vi "data_load_display_trend_fft_mea_coll_v3.vi"() -> ()   [LabVIEW 2020]
uses:
  <vilib>/Analysis/2dsp.llb/Real FFT.vi
  <vilib>/Utility/file.llb/Read Delimited Spreadsheet (DBL).vi
  <vilib>/Utility/file.llb/Read Delimited Spreadsheet (string).vi
  <vilib>/ptbypt/NI_PtbyPt.lvlib
  <vilib>/Analysis/NI_AALPro.lvlib
  <vilib>/rvi/Analysis/host/Public/NI_FpgaMspHost.lvlib
panel:
  out "Waveform Graph":dbl[][](graph)
  out "XY Graph":cluster{dbl[], dbl[]}(graph)
  out "restored signal":dbl[](array[numeric])
  out "plot restored signal":dbl[](graph)
  out "ploted signal from each selected frequency":dbl[][](graph)
  out "signal from each selected frequency":dbl[][](array[numeric])
  out "phase":dbl[](array[numeric])
  out "magnitude":dbl[](array[numeric])
  out "phase":dbl format="%0.2f"
  out "magnitude":dbl format="%0.2f"
  out "magnitude plot":dbl[](graph)
  out "phase plot":dbl[](graph)
  out "magnitudes":dbl[](array[numeric])
  out "phasees":dbl[](array[numeric])
  out "df (Hz)":dbl
  out "size(s)":i32
  out "xf (frequency)":dbl[](array[numeric])
  in  "decimating factor":i32=3
  out "xf (sample Vs frequency )":dbl[][](array[numeric]) format="%#20_5g"
  out "Imaginary values":dbl[](array[numeric])
  out "real  values":dbl[](array[numeric])
  out "real plot":dbl[](graph)
  out "imaginary plot":dbl[](graph)
  out "Time Domain sequence":cluster{i32, dbl, dbl[]}(graph)
  out "Frequency Interval: delta(f)":dbl
  out "Spectrum plot":cluster{i32, dbl, "spectrum out":dbl[]}(graph)
  out "Remove trend":cluster{"all rows":dbl[], dbl[]}(graph)
  out "Time vs Acceleration  find trend graph":T1(graph)
  out "array w/ subset deleted":dbl[][](array[numeric])
  out "first row":string[][](array[string])
  out "time":dbl[](array[numeric])
  out "Acceleration":dbl[](array[numeric])
  out "Time vs Acceleration graph":cluster{"all rows":dbl[], "all rows":dbl[]}(graph)
  out "stripped path":path
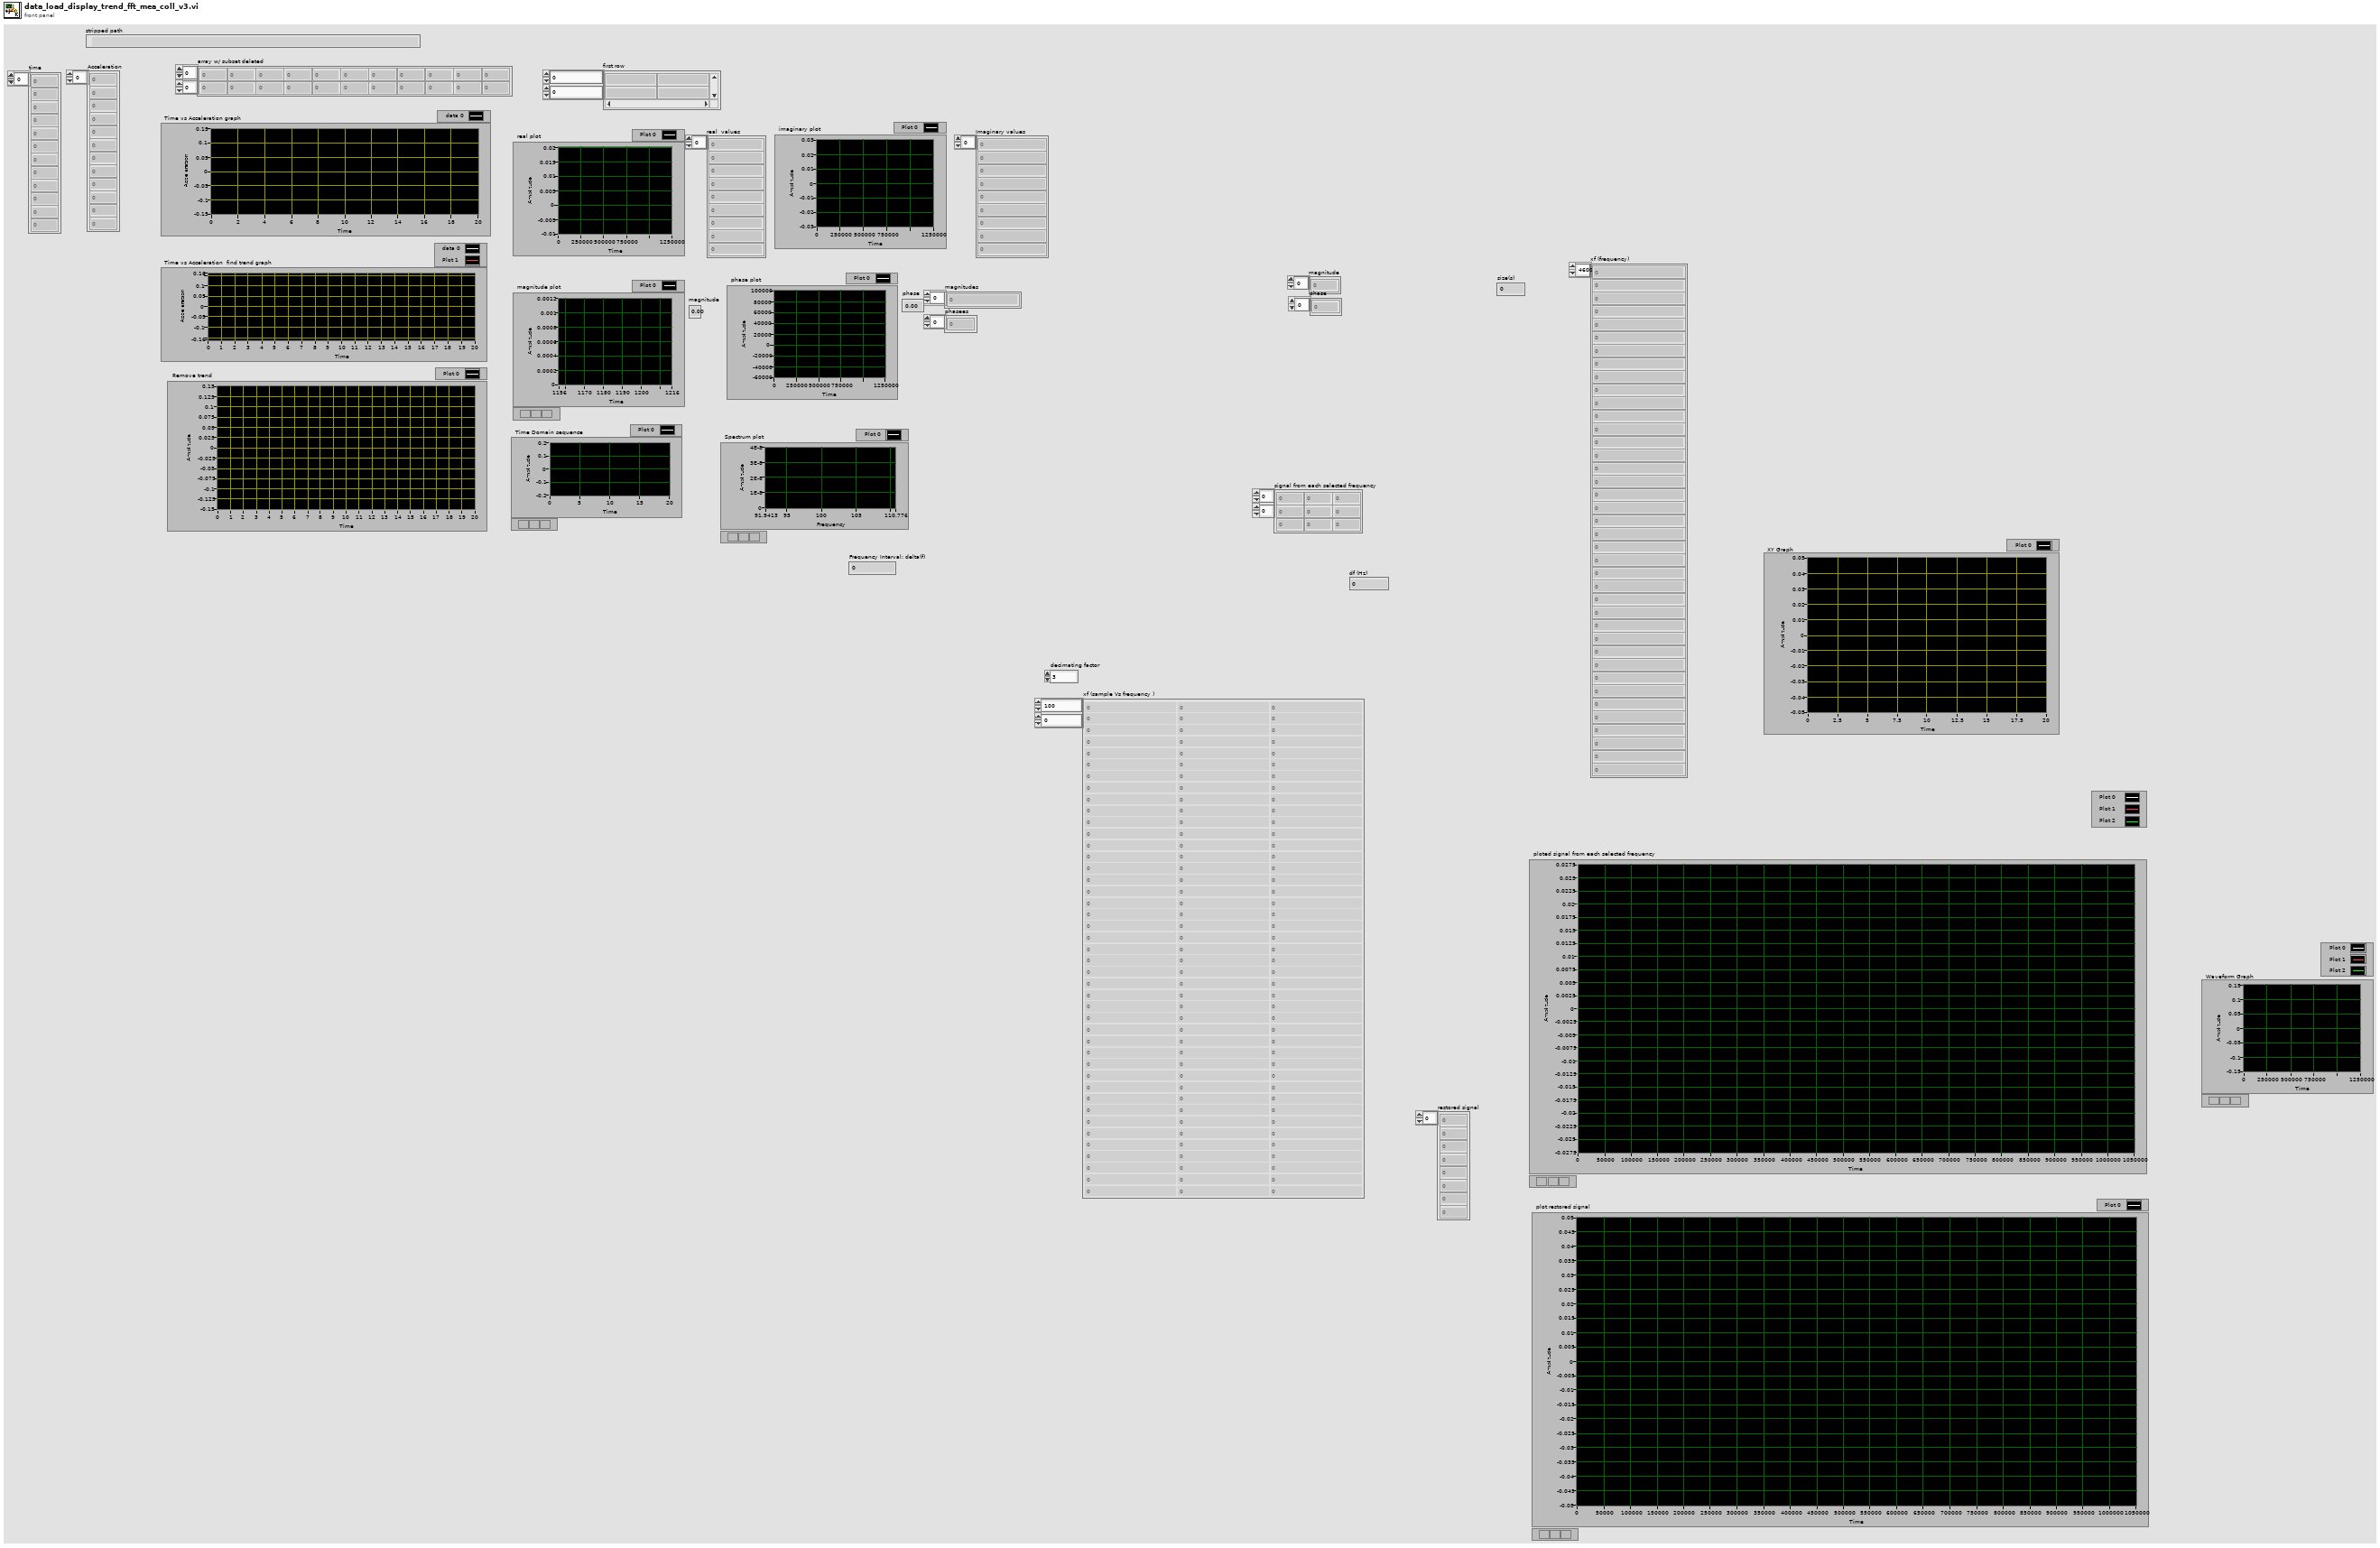
[diagram p1: front panel]
types:
  T1 = cluster{"all rows":dbl[], "Best Linear Fit":dbl[]}
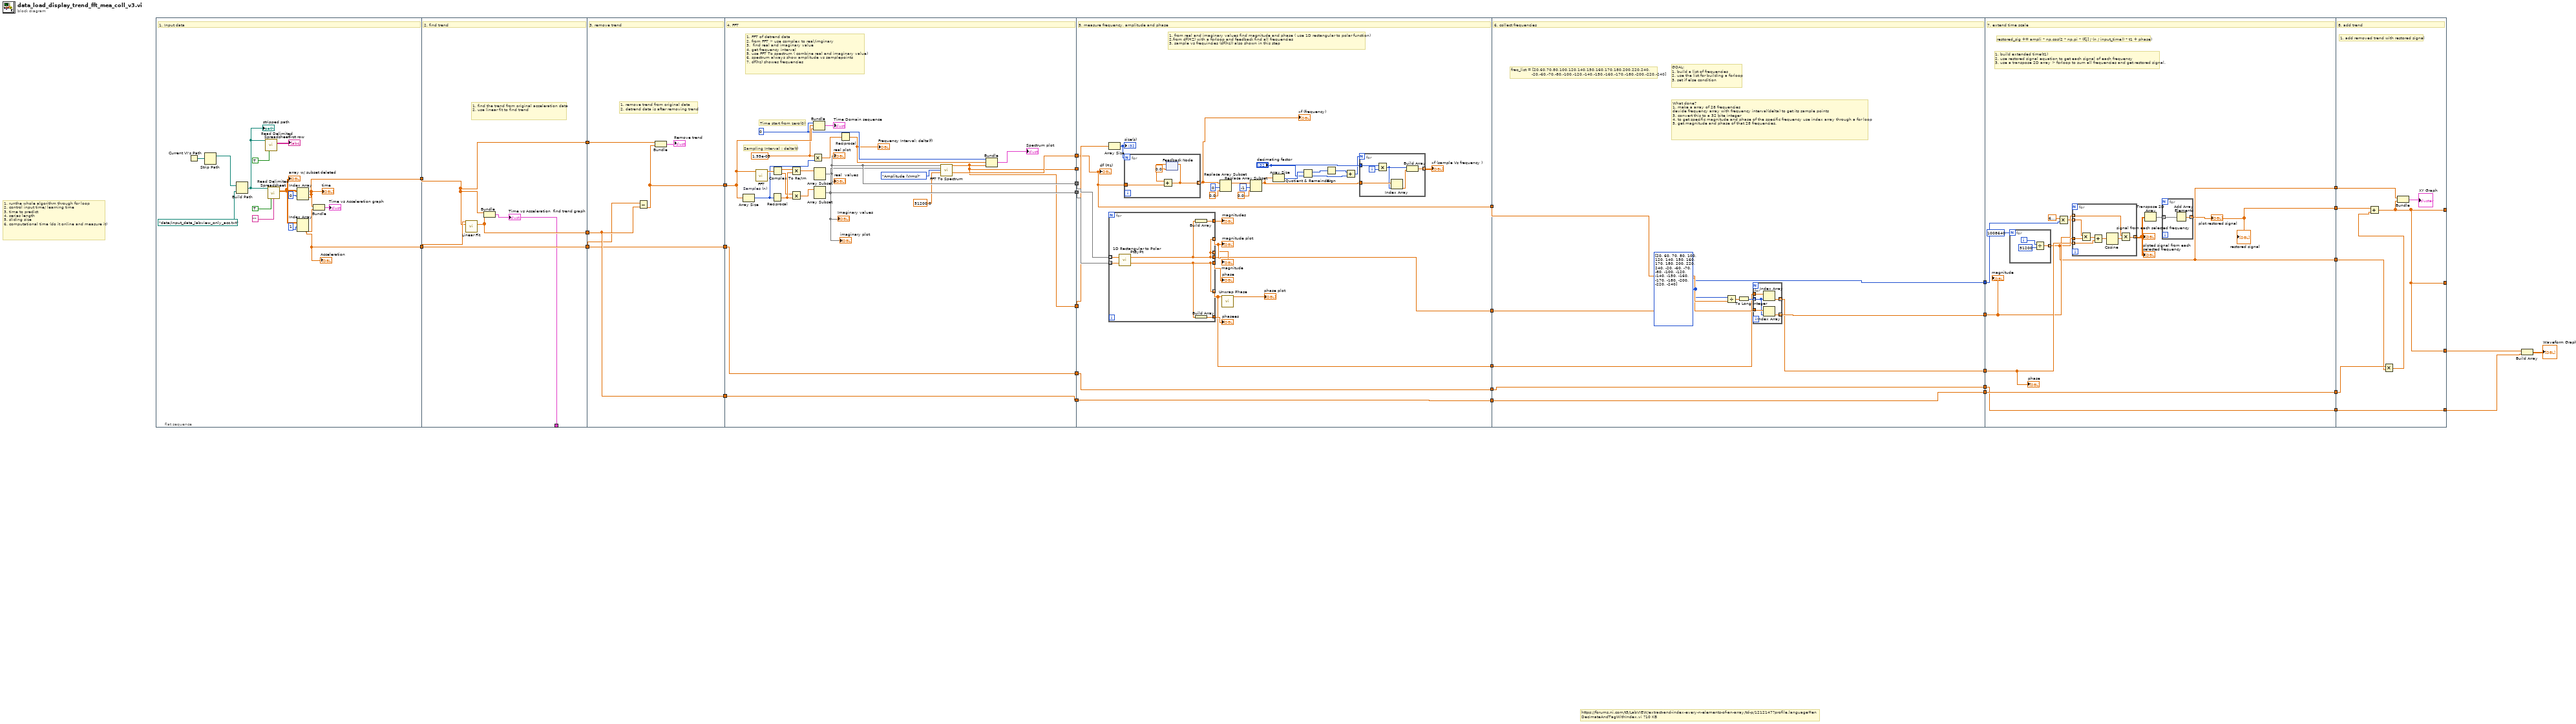
[diagram p0: block diagram]
diagram:
  # "1. runthe whole algorithm through for loop \n2. control input time/ learning time\n3. time to predict\n4. series length\n5. sliding size\n6. computational time (do it online and measure it)"
  # "https://forums.ni.com/t5/LabVIEW/extract-and-index-every-n-elements-of-an-array/td-p/1212147?profile.language=en\nDecimateAndTagWithIndex.vi ?10 KB"
  n1 = flat-sequence {
    tunnel: [w35] -> w33
    tunnel: [w34] -> w32
    tunnel: w33 -> [w50]
    tunnel: [w51] -> w31
    tunnel: [w50] -> w30
    tunnel: [w49] -> w29
    tunnel: w32 -> [w49]
    tunnel: [w48] -> _
    tunnel: w31 -> [w53]
    tunnel: w30 -> [w52]
    tunnel: w29 -> [w56]
    tunnel: [w55] -> w28
    tunnel: [w53] -> w27
    tunnel: [w52] -> w8
    tunnel: w28 -> [w72]
    tunnel: [w69] -> w26
    tunnel: [w68] -> w25
    tunnel: [w60] -> w24
    tunnel: [w61] -> w23
    tunnel: [w60] -> w22
    tunnel: [w58] -> w21
    tunnel: w27 -> [w58]
    tunnel: w8 -> [w57]
    tunnel: [w57] -> w7
    tunnel: w26 -> [w106]
    tunnel: w25 -> [w105]
    tunnel: w24 -> [_]
    tunnel: w23 -> [w84]
    tunnel: w22 -> [w99]
    tunnel: [w84] -> w20
    tunnel: [w83] -> w19
    tunnel: [w81] -> w18
    tunnel: [w80] -> w17
    tunnel: w21 -> [w80]
    tunnel: w7 -> [w79]
    tunnel: [w79] -> w6
    tunnel: w20 -> [w132]
    tunnel: [w129] -> w16
    tunnel: w19 -> [w128]
    tunnel: w18 -> [w127]
    tunnel: [w126] -> w15
    tunnel: [w125] -> w14
    tunnel: [w124] -> w13
    tunnel: w17 -> [w124]
    tunnel: w6 -> [w123]
    tunnel: [w123] -> w5
    tunnel: w16 -> [w147]
    tunnel: w15 -> [w148]
    tunnel: w14 -> [w143]
    tunnel: [w141] -> w12
    tunnel: [w140] -> w11
    tunnel: w13 -> [w140]
    tunnel: [w139] -> w10
    tunnel: [w139] -> w9
    tunnel: w5 -> [w138]
    tunnel: [w138] -> w4
    tunnel: w12 -> [w170]
    tunnel: w11 -> [w168]
    tunnel: w10 -> [w169]
    tunnel: w9 -> [w167]
    tunnel: [w164] -> _
    tunnel: [w165] -> w2
    tunnel: w4 -> [w165]
    tunnel: [w164] -> _
    tunnel: [w164] -> w3
    frame #0 {
      # "1. Input data"
      n2 = Current VI's Path() -> (path=w39:path)
      n3 = Strip Path(path=w39) -> (stripped path=w38:path)  [unwired: 1 out]
      n4 = Build Path(base path=w38, name or relative path=path "data/input_data_labview_only_acc.txt") -> (appended path=w36:path)
      "stripped path" <- w36
      n5 = call-poly <vilib>:"Read Delimited Spreadsheet.vi"("file path (dialog if empty)"=w36, "transpose? (F)"=TRUE) -> ("all rows"=→"first row":string[][])  [unwired: 8 in, 5 out]
      n6 = call-poly <vilib>:"Read Delimited Spreadsheet.vi"("file path (dialog if empty)"=w36, "transpose? (F)"=TRUE, "delimiter (\\t)"="" ("delimiter (\\t)")) -> ("all rows"=w41:dbl[][])  [unwired: 7 in, 5 out]
      "array w/ subset deleted" <- w41
      n7 = Index Array(array=w41, index (row)=0) -> (element=w34:dbl[])  [unwired: 1 in]
      "time" <- w34
      n8 = Index Array(array=w41, index (row)=1) -> (element=w35:dbl[])  [unwired: 1 in]
      "Acceleration" <- w35
      n9 = Bundle("all rows"=w34, "all rows"=w35) -> (→"Time vs Acceleration graph":cluster{"all rows":dbl[], "all rows":dbl[]})  [unwired: 1 in]
    }
    frame #1 {
      # "1. find the trend from original acceleration data\n2. use linear fit to find trend"
      # "2. find trend"
      n10 = call <vilib>:"Linear Fit.vi"("Y"=w50, "X"=w49) -> ("Best Linear Fit"=w51:dbl[])  [unwired: 9 in, 4 out]
      n11 = Bundle("all rows"=w49, "Best Linear Fit"=w51) -> (w48:T1)  [unwired: 1 in]
      "Time vs Acceleration  find trend graph" <- w48
    }
    frame #2 {
      # "1. remove trend from original data\n2. detrend data is after removing trend"
      # "3. remove trend"
      n12 = Subtract(x=w52, y=w53) -> (x-y=w55:dbl[])
      n13 = Bundle("all rows"=w56, w55) -> (→"Remove trend":cluster{"all rows":dbl[], dbl[]})  [unwired: 1 in]
    }
    frame #3 {
      w70 = 1.95e-05
      w66 = 0
      # "1. FFT of detrend data\n2. from FFT > use complex to real/imginary\n3.  find real and imaginary value\n4. get frequency interval\n5. use FFT To spectrum ( combine real and imaginary value)\n6. spectrum always show amplitude vs samplepoints\n7. df(hz) showes frequencies"
      # "Sampling Interval : delta(t)"
      # "Time start from zero(0)"
      # "4. FFT"
      n14 = Array Size "Samples (n)"(array=w72) -> (size(s)=w62:i32)
      n15 = call-poly <vilib>:"FFT.vi"("X"=w72) -> ("FFT {X}"=w64:cdb[])  [unwired: 9 in, 1 out]
      n16 = Reciprocal(x=w62) -> (1/x=w78:dbl)
      n17 = Complex To Re/Im(x + iy=w64) -> (x=w77:dbl[], y=w76:dbl[])
      n18 = Multiply(x=w77, y=w78) -> (x*y=w74:dbl[])
      n19 = Multiply(x=w76, y=w78) -> (x*y=w75:dbl[])
      n20 = Multiply(x=w70, y=w62) -> (x*y=w73:dbl)
      n21 = Bundle(w66, w70, w72) -> (→"Time Domain sequence":cluster{i32, dbl, dbl[]})  [unwired: 1 in]
      n22 = Array Subset(array=w74) -> (w69:dbl[])  [unwired: 2 in]
      "real  values" <- w69
      "real plot" <- w69
      n23 = Array Subset(array=w75) -> (w68:dbl[])  [unwired: 2 in]
      "Imaginary values" <- w68
      "imaginary plot" <- w68
      n24 = Reciprocal(x=w73) -> (1/x=w63:dbl)
      "Frequency Interval: delta(f)" <- w63
      n25 = call <vilib>:"FFT To Spectrum.vi"("real FFT data"=w69, "imaginary FFT data"=w68, "spectrum type"=enum8{"Power (Vrms^2)", "Amplitude (Vrms)"}."Amplitude (Vrms)", "sample rate (S/s)"=51200.0) -> ("spectrum out"=w60:dbl[], "df (Hz)"=w61:dbl)  [unwired: 9 in, 1 out]
      n26 = Bundle(w66, w63, "spectrum out"=w60) -> (→"Spectrum plot":cluster{i32, dbl, "spectrum out":dbl[]})  [unwired: 1 in]
    }
    frame #4 {
      # "1. from real and imaginary values find magnitude and phase ( use 1D rectangular to polar function)\n2.from df(HZ) with a forloop and feedback find all frequencies \n3. sample vs frequincies (df(hz)) also shown in this step"
      # "5. measure frequency, amplitude and phase"
      n27 = Array Size(array=w99) -> (size(s)=w100:i32)
      "size(s)" <- w100
      n28 = for {
        tunnel: w106 -> [w122] mode=indexing
        tunnel: w105 -> [w121] mode=indexing
        tunnel: [w120] -> w104
        tunnel: [w117] -> w82
        tunnel: [w117] -> w83 mode=indexing
        tunnel: [w120] -> w81 mode=indexing
        tunnel: [w119] -> w103
        tunnel: [w118] -> w102
        tunnel: [w117] -> _ mode=indexing
        n29 = call <vilib>:"1D Rectangular to Polar PtByPt.vi"("y"=w121, "x"=w122) -> ("phase"=w120:dbl, "magnitude"=w117:dbl)
        n30 = Build Array(w117) -> (w119:dbl[])
        n31 = Build Array(w120) -> (w118:dbl[])
      }
      "phase" <- w104
      "magnitude" <- w82
      "magnitude plot" <- w83
      "magnitudes" <- w103
      "phasees" <- w102
      n32 = for {
        N: w100 -> [_]
        tunnel: w84 -> [w115]
        tunnel: [w113] -> w85 mode=indexing
        n33 = feedback #1(0.0) -> (w116:dbl)
        n34 = Add(x=w116, y=w115) -> (x+y=w113:dbl)
        n35 = feedback-in #1(w113) -> ()
      }
      "xf (frequency)" <- w85
      n36 = Replace Array Subset(array=w85, new element=0.0 ("new element/subarray"), index=0) -> (w90:dbl[])
      n37 = call <vilib>:"Unwrap Phase.vi"("Phase"=w81) -> ("Unwrapped Phase"=→"phase plot":dbl[])  [unwired: 9 in, 1 out]
      n38 = Replace Array Subset(array=w90, new element=0.0 ("new element/subarray"), index=-1) -> (w87:dbl[])
      n39 = Array Size(array=w87) -> (size(s)=w98:i32)
      n40 = Quotient & Remainder(x=w98, y="decimating factor") -> (x-y*floor(x/y)=w96:i32, floor(x/y)=w95:i32)
      n41 = Sign(1:w96) -> (0:w94:i32)
      n42 = Add(x=w94, y=w95) -> (x+y=w93:i32)
      n43 = for {
        N: w93 -> [_]
        tunnel: w87 -> [w112]
        tunnel: [w109] -> w86 mode=indexing
        tunnel: "decimating factor" -> [w108]
        i -> [w111]
        n44 = Multiply(x=w108, y=w111) -> (x*y=w107:i32)
        n45 = Index Array(array=w112, index=w107) -> (element=w110:dbl)
        n46 = Build Array(w107, w110) -> (w109:dbl[])
      }
      "xf (sample Vs frequency )" <- w86
      "df (Hz)" <- w84
    }
    frame #5 {
      w125 = i32[] [20, 60, 70, 80, 100, 120, 140, 150, 160, 170, 180, 200, 220, 240, -20, -60, -70, -80, -100, -120, -140, -150, -160, -170, -180, -200, -220, -240]
      # "What done?\n1. make a array of 28 frequencies\ndevide frequency array with frequency interval(delta) to get its sample points\n3. convert this to a 32 bite integer\n4. to get specific magnitude and phase of the specific frequency use index array through a for loop\n5. get magnitude and phase of that 28 frequencies."
      # "freq_list = [20,60,70,80,100,120,140,150,160,170,180,200,220,240,\n                -20,-60,-70,-80,-100,-120,-140,-150,-160,-170,-180,-200,-220,-240]"
      # "GOAL:\n1. build a list of frequencies\n2. use the list for building a forloop\n3. set if else condition"
      # "6. collect frequencies"
      n47 = Divide(x=w125, y=w132) -> (x/y=w131:dbl[])
      n48 = To Long Integer(number=w131) -> (32bit integer=w130:i32[])
      n49 = for {
        tunnel: w130 -> [w135] mode=indexing
        tunnel: w128 -> [w137]
        tunnel: [w136] -> w129 mode=indexing
        tunnel: w127 -> [w134]
        tunnel: [w133] -> w126 mode=indexing
        n50 = Index Array(array=w134, index=w135) -> (element=w133:dbl)
        n51 = Index Array(array=w137, index=w135) -> (element=w136:dbl)
      }
    }
    frame #6 {
      # "1. build extended time(t1)\n2. use restored signal equation to get each signal of each frequency\n3. use a transpose 2D array > forloop to sum all frequencies and get restored signal."
      # "restored_sig += ampli * np.cos(2 * np.pi * (f[j] / (n / input_time)) * t1 + phase)"
      # "7. extend time scale"
      n52 = for {
        N: 1008640 -> [_]
        tunnel: [w152] -> w139 mode=indexing
        i -> [w154]
        n53 = Divide(x=w154, y=51200) -> (x/y=w152:dbl)
      }
      n54 = Multiply(x=6.283185307179586, y=w143) -> (x*y=w142:dbl[])
      n55 = for {
        tunnel: w139 -> [w162]
        tunnel: w148 -> [w160] mode=indexing
        tunnel: w147 -> [w159] mode=indexing
        tunnel: [w158] -> w146 mode=indexing
        tunnel: w142 -> [w157] mode=indexing
        n56 = Multiply(x=w157, y=w162) -> (x*y=w161:dbl[])
        n57 = Add(x=w161, y=w160) -> (x+y=w156:dbl[])
        n58 = Cosine(x=w156) -> (cos(x)=w155:dbl[])
        n59 = Multiply(x=w159, y=w155) -> (x*y=w158:dbl[])
      }
      "signal from each selected frequency" <- w146
      "ploted signal from each selected frequency" <- w146
      n60 = Transpose 2D Array(2D array=w146) -> (transposed array=w145:dbl[][])
      n61 = for {
        tunnel: w145 -> [w151] mode=indexing
        tunnel: [w150] -> w141 mode=indexing
        n62 = Add Array Elements(numeric array=w151) -> (sum=w150:dbl)
      }
      "plot restored signal" <- w141
      "restored signal" <- w141
      "magnitude" <- w147
      "phase" <- w148
    }
    frame #7 {
      # "1. add removed trend with restored signal"
      # "8. add trend"
      n63 = Multiply(x=w168, y=w167) -> (x*y=w166:dbl[])
      n64 = Add(x=w170, y=w166) -> (x+y=w164:dbl[])
      n65 = Bundle(w169, w164) -> (→"XY Graph":cluster{dbl[], dbl[]})  [unwired: 1 in]
    }
  }
  n66 = Build Array(w3, w2) -> (→"Waveform Graph":dbl[][])
